vi "BRig_dataTrial_iError.vi"() -> (2 "output_iError":i32)   [LabVIEW 2014]
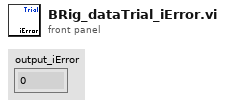
[diagram p1: front panel]
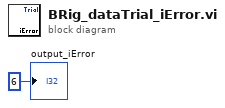
[diagram p0: block diagram]
diagram:
  "output_iError" <- 6 ("output_iBlock")
